vi "UART Close.vi"(8 "error in (no error)":errorcluster, 11 "VISA resource name in":refnum<visa-resource-name>) -> (0 "error out":errorcluster)   [LabVIEW 2021, in "UART.lvlib"]
doc: "Closes a device session or event object."
uses:
  <vilib>/myRIO/Instrument Drivers/Onboard IO/UART/UART.lvlib
  <vilib>/myRIO/Common/Instrument Driver Framework/ELVIS III v1.0/UART/vis/ELVIS III v1.0 Unreserve UART.vi
  <vilib>/myRIO/Common/Instrument Driver Framework/ELVIS III v1.0/UART/vis/ELVIS III v1.0 Build MUX Configuration UART.vi
  <vilib>/myRIO/Common/Instrument Driver Framework/Utilities/vis/FPGA Ref Manager.vi
  <vilib>/myRIO/Common/Instrument Driver Framework/ELVIS III v1.0/UART/vis/ELVIS III v1.0 Configure UART.vi
  <vilib>/myRIO/Common/Instrument Driver Framework/ELVIS III v1.0/Resource Manager/vis/ELVIS III v1.0 Unreserve Channel List.vi
  <vilib>/myRIO/Common/Instrument Driver Framework/myRIO v1.0/myRIO v1.0 Close.vi
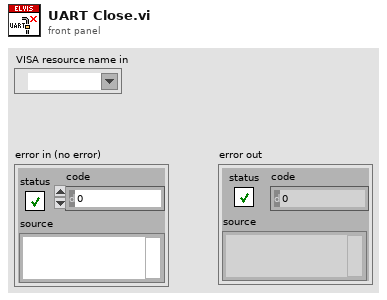
[diagram p1: front panel]
types:
  T1 = typedef "Hardware Version Enum.ctl" = enum16{"Unknown", "myRIO-1900", "myRIO-1950", "roboRIO", "NI ELVIS RIO CM", "ELVIS III"}
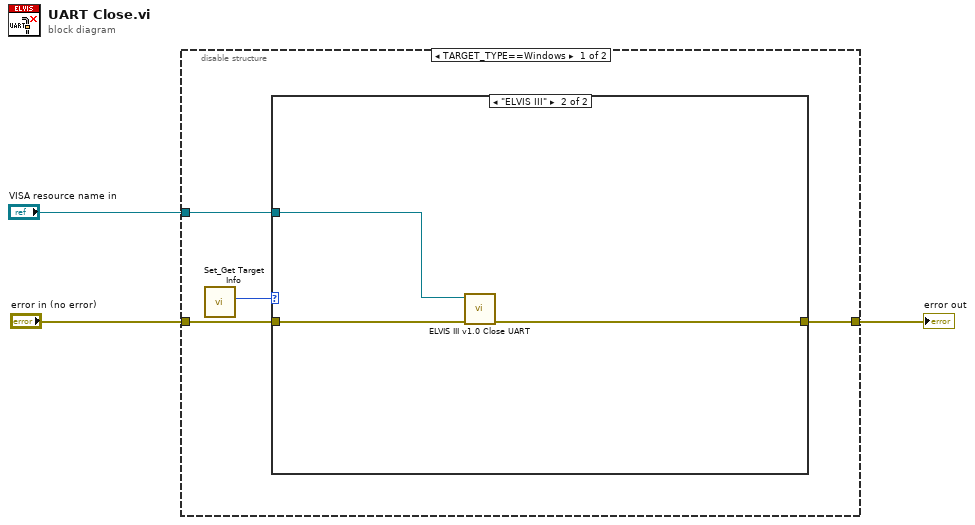
[diagram p0: block diagram]
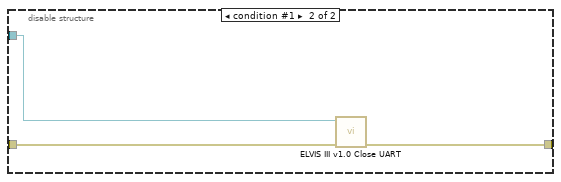
[diagram p4: hidden frame]
diagram:
  n1 = disable-structure shown="TARGET_TYPE==Windows" {
    disable-tunnel: "VISA resource name in" -> [w7 w14]
    disable-tunnel: "error in (no error)" -> [w5 w12]
    disable-tunnel: [w6 w13] -> w1
    frame condition #0 (active) {
      n2 = call <vilib>:"Set_Get Target Info.vi"() -> ("Hardware Version"=w4:T1)  [unwired: 9 in, 2 out]
      n3 = case shown="\"ELVIS III\"" w4 {
        tunnel: w7 -> [_ w9]
        tunnel: w5 -> [w8 w11]
        tunnel: [w8 w10] -> w6
        frame "Unknown", Default {
        }
        frame "ELVIS III" {
          n4 = call <vilib>:"ELVIS III v1.0 Close UART.vi"("error in (no error)"=w11, "VISA resource name in"=w9) -> ("error out"=w10:errorcluster)  [unwired: 9 in]
        }
      }
    }
    frame condition #1 {
      n5 = disable-structure shown="Default" {
        disable-tunnel: w14 -> [_ w18]
        disable-tunnel: [w15 w16] -> w13
        disable-tunnel: w12 -> [w15 w17]
        frame condition #0 (active) {
        }
        frame condition #1 {
          n6 = call <vilib>:"ELVIS III v1.0 Close UART.vi"("error in (no error)"=w17, "VISA resource name in"=w18) -> ("error out"=w16:errorcluster)  [unwired: 9 in]
        }
      }
    }
  }
  "error out" <- w1
